vi "Filter Nodes by Name.vi"() -> ()   [LabVIEW 2021, in "Tree Map.lvlib"]
doc: "<b>Author:</b> Piotr Kruczkowski <PrimaryKey>\n<b>License:</b> NewBSD\n\nCopyright (c) 2019, National Instruments\nAll rights reserved.\n\nRedistribution and use in source and binary forms, with or without\nmodification, are permitted provided that the following conditions are met:\n1. Redistributions of source code must retain the above copyright\n notice, this list of conditions and the following disclaimer.\n2. Redistributions in binary form must reproduce the above copyright\n notice, this list of conditions and the following disclaimer in the\n documentation and/or other materials provided with the distribution.\n3. Neither the name of National Instruments nor the\n names of its contributors may be used to endorse or promote products\n derived from this software without specific prior written permission.\n\nTHIS SOFTWARE IS PROVIDED BY National Instruments ''AS IS'' AND ANY\nEXPRESS OR IMPLIED WARRANTIES, INCLUDING, BUT NOT LIMITED TO, THE IMPLIED\nWARRANTIES OF MERCHANTABILITY AND FITNESS FOR A PARTICULAR PURPOSE ARE\nDISCLAIMED. IN NO EVENT SHALL National Instruments BE LIABLE FOR ANY\nDIRECT, INDIRECT, INCIDENTAL, SPECIAL, EXEMPLARY, OR CONSEQUENTIAL DAMAGES\n(INCLUDING, BUT NOT LIMITED TO, PROCUREMENT OF SUBSTITUTE GOODS OR SERVICES;\nLOSS OF USE, DATA, OR PROFITS; OR BUSINESS INTERRUPTION) HOWEVER CAUSED AND\nON ANY THEORY OF LIABILITY, WHETHER IN CONTRACT, STRICT LIABILITY, OR TORT\n(INCLUDING NEGLIGENCE OR OTHERWISE) ARISING IN ANY WAY OUT OF THE USE OF THIS\nSOFTWARE, EVEN IF ADVISED OF THE POSSIBILITY OF SUCH DAMAGE."
uses:
  <vilib>/National Instruments/Tree Map/Tree Map.lvlib
  <vilib>/National Instruments/Tree Map/Utility/Join Strings Tree.vi
  <vilib>/National Instruments/Tree Map/SubVIs/TM Head and Tail.vi
  <vilib>/National Instruments/Tree Map/SubVIs/TM Init and Last.vi
  <vilib>/National Instruments/Tree Map/Utility/Split String Tree.vi
panel:
  in  "Name Filter":string="Value"
  out "Filtered Paths":string[](array[string])=["\\Config\\Info\\Value", "\\Config\\Info\\Value_000000", "\\Config\\Info\\Value_000001"]
  out "Tree XML":string="<Config>\n    <Info>\n        <Value Attr=\"Foo\" Attr2=\"Bar\">0</Value>\r\n        <Value Attr=\"Foo\" Attr2=\"Bar\">1</Value>\r\n        <Value Attr=\"Foo\" Attr2=\"Bar\">2</Value>\n    </Info>\n</Config>"
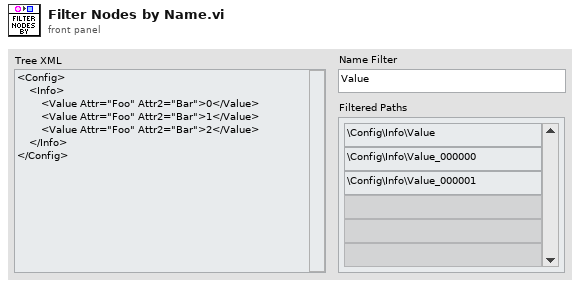
[diagram p1: front panel]
types:
  T1 = typedef "Tree Map.lvlib/Tree Map Data.ctl" = map{string, cluster{"Child Paths Set":set{string}, "Name":string, "Data":string, "Attributes":map{string, string}}}
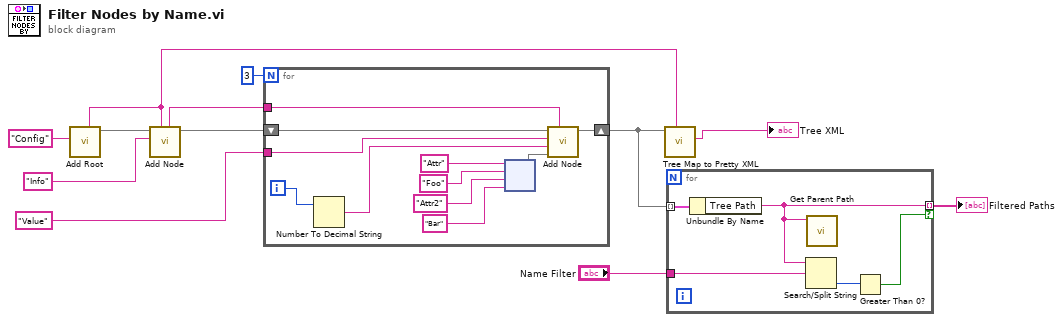
[diagram p0: block diagram]
diagram:
  n1 = call <vilib>:"Add Root.vi"("New Root Name"="Config") -> ("Tree Map Out"=w11:T1, "Root Path"=w2:string)  [unwired: 9 in]
  n2 = call <vilib>:"Add Node.vi"("Parent Path"=w2, "New Node Name"="Info" ("New Branch Name"), "Tree Map In"=w11) -> ("Tree Map Out"=w4:T1, "New Node Path"=w6:string)  [unwired: 6 in, 1 out]
  n3 = for {
    N: 3 -> [_]
    shift-right: [w19] -> w3
    shift-left: w4 -> [w23]
    tunnel: w6 -> [w21]
    tunnel: "Value" ("format string") -> [w13]
    i -> [w22]
    n4 = Number To Decimal String(number=w22) -> (decimal integer string=w20:string)  [unwired: 1 in]
    n5 = node("Attr" ("key"), "Foo" ("key"), "Attr2" ("key"), "Bar" ("key")) -> (w16:map{string, string})
    n6 = call <vilib>:"Add Node.vi"("Parent Path"=w21, "Attributes"=w16, "Data"=w20, "New Node Name"=w13, "Tree Map In"=w23) -> ("Tree Map Out"=w19:T1)  [unwired: 4 in, 2 out]
  }
  n7 = call <vilib>:"Tree Map to Pretty XML.vi"("Root Path"=w2, "Tree Map In"=w3) -> ("Pretty XML"=→"Tree XML":string)  [unwired: 8 in, 1 out]
  n8 = for {
    tunnel: w3 -> [w28] mode=indexing
    tunnel: "Name Filter" -> [w27]
    tunnel: [w26] -> w9 mode=indexing if=w24
    n9 = Unbundle By Name(w28) -> ("Tree Path"=w26:string)
    n10 = Search/Split String(string=w26, search string/char (-)=w27) -> (offset of match=w25:i32)  [unwired: 1 in, 2 out]
    n11 = call <vilib>:"Get Parent Path.vi"("Node Path"=w26) -> ()  [unwired: 8 in, 3 out]
    n12 = Greater Than 0?(x=w25) -> (x > 0?=w24:bool)
  }
  "Filtered Paths" <- w9
